vi "Odom_Begin.vi"   [LabVIEW 2020]
uses:
  <vilib>/Rock Robotics/WPI/ThirdParty/JAS_Junk/TrajLib/Rotation2d_CreateAngle.vi
  <vilib>/Rock Robotics/WPI/ThirdParty/JAS_Junk/TrajLib/Translation2d_Create.vi
  Robot Global Data.vi
  <vilib>/Rock Robotics/WPI/ThirdParty/JAS_Junk/TrajLib/Trajectory_Library.lvlib
types:
  T1 = typedef "Trajectory_Library.lvlib/ROTATION2D.ctl" = cluster{"VALUE":dbl, "COS":dbl, "SIN":dbl}
  T2 = typedef "Trajectory_Library.lvlib/SWERVE_DRIVE_MODULE_STATE.ctl" = cluster{"Speed":dbl, "Angle":T1}
  T3 = typedef "Trajectory_Library.lvlib/SWERVE_DRIVE_MODULE_POSITION.ctl" = cluster{"Distance":dbl, "Angle":T1, "P":bool}
  T4 = typedef "Trajectory_Library.lvlib/POSE2D.ctl" = cluster{"TRANSLATION":T5, "ROTATION":T1}
  T5 = typedef "Trajectory_Library.lvlib/TRANSLATION2D.ctl" = cluster{"X":dbl, "Y":dbl}
  T6 = typedef "Trajectory_Library.lvlib/SWERVE_DRIVE_ODOMETRY.ctl" = cluster{"POSE":T4, "GyroOffset":T1, "PreviousAngle":T1, "PrevModulePositions":T3[], "NumModules":i32}
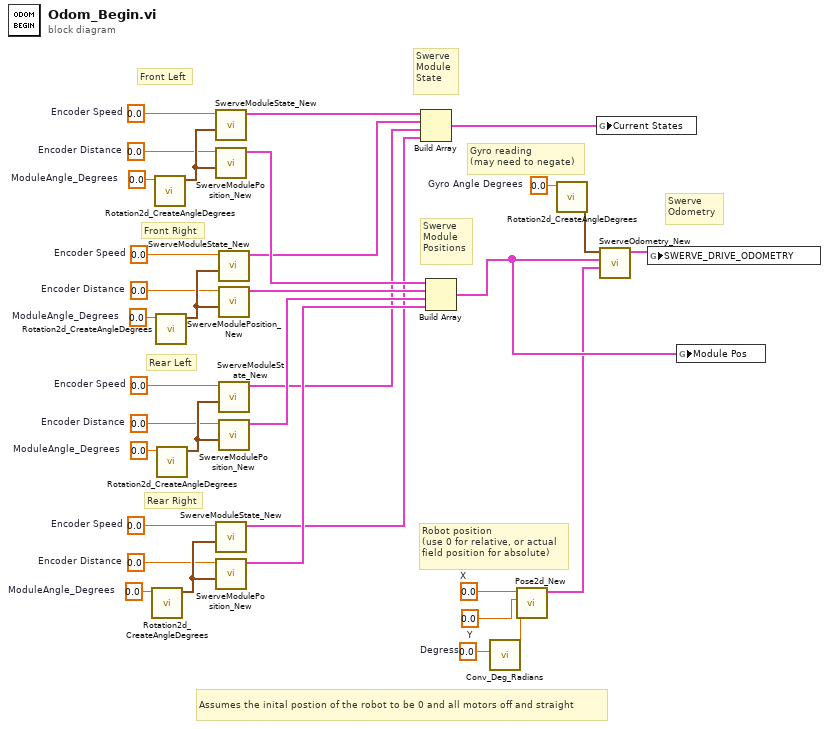
[diagram p0: block diagram]
diagram:
  w18 = 0.0  # Encoder Distance
  w17 = 0.0  # Encoder Distance
  w16 = 0.0  # Encoder Distance
  w14 = 0.0  # Encoder Distance
  w10 = 0.0  # ModuleAngle_Degrees
  w9 = 0.0  # Encoder Speed
  w8 = 0.0  # ModuleAngle_Degrees
  w7 = 0.0  # Encoder Speed
  w6 = 0.0  # ModuleAngle_Degrees
  w5 = 0.0  # Encoder Speed
  w3 = 0.0  # ModuleAngle_Degrees
  w2 = 0.0  # Encoder Speed
  w32 = 0.0  # Degress
  w31 = 0.0  # X
  w30 = 0.0  # Y
  w27 = 0.0  # Gyro Angle Degrees
  # "Assumes the inital postion of the robot to be 0 and all motors off and straight"
  # "Swerve\nModule\nPositions"
  # "Front Left"
  # "Swerve\nModule\nState"
  # "Rear Right"
  # "Rear Left"
  # "Front Right"
  # "Swerve\nOdometry"
  # "Robot position\n(use 0 for relative, or actual \nfield position for absolute)"
  # "Gyro reading\n(may need to negate)"
  n1 = call <vilib>:"Rotation2d_CreateAngleDegrees.vi"("Angle_Degrees"=w10) -> ("ROTATION"=w25:T1)  [unwired: 10 in]
  n2 = call <vilib>:"Rotation2d_CreateAngleDegrees.vi"("Angle_Degrees"=w3) -> ("ROTATION"=w22:T1)  [unwired: 10 in]
  n3 = call <vilib>:"Rotation2d_CreateAngleDegrees.vi"("Angle_Degrees"=w6) -> ("ROTATION"=w23:T1)  [unwired: 10 in]
  n4 = call <vilib>:"Rotation2d_CreateAngleDegrees.vi"("Angle_Degrees"=w8) -> ("ROTATION"=w24:T1)  [unwired: 10 in]
  n5 = call <vilib>:"SwerveModuleState_New.vi"("ROTATION"=w22, "Speed"=w2) -> ("SWERVE_DRIVE_MODULE_STATE"=w4:T2)  [unwired: 9 in]
  n6 = call <vilib>:"SwerveModulePosition_New.vi"("ROTATION"=w22, "Distance"=w14) -> ("SWERVE_DRIVE_MODULE_POSITION"=w15:T3)  [unwired: 9 in]
  n7 = call <vilib>:"SwerveModuleState_New.vi"("ROTATION"=w25, "Speed"=w9) -> ("SWERVE_DRIVE_MODULE_STATE"=w13:T2)  [unwired: 9 in]
  n8 = call <vilib>:"SwerveModulePosition_New.vi"("ROTATION"=w25, "Distance"=w18) -> ("SWERVE_DRIVE_MODULE_POSITION"=w21:T3)  [unwired: 9 in]
  n9 = call <vilib>:"SwerveModuleState_New.vi"("ROTATION"=w23, "Speed"=w5) -> ("SWERVE_DRIVE_MODULE_STATE"=w11:T2)  [unwired: 9 in]
  n10 = call <vilib>:"SwerveModulePosition_New.vi"("ROTATION"=w23, "Distance"=w16) -> ("SWERVE_DRIVE_MODULE_POSITION"=w19:T3)  [unwired: 9 in]
  n11 = call <vilib>:"SwerveModuleState_New.vi"("ROTATION"=w24, "Speed"=w7) -> ("SWERVE_DRIVE_MODULE_STATE"=w12:T2)  [unwired: 9 in]
  n12 = call <vilib>:"SwerveModulePosition_New.vi"("ROTATION"=w24, "Distance"=w17) -> ("SWERVE_DRIVE_MODULE_POSITION"=w20:T3)  [unwired: 9 in]
  n13 = Build Array(w4, w11, w12, w13) -> (w1:T2[])
  n14 = Build Array(w15, w19, w20, w21) -> (w34:T3[])
  n15 = call <vilib>:"Conv_Deg_Radians.vi"("Degress"=w32) -> ("Radians"=w29:dbl)  [unwired: 10 in]
  n16 = call <vilib>:"Pose2d_New.vi"("Heading"=w29, "Y"=w30, "X"=w31) -> ("out POSe"=w33:T4)  [unwired: 8 in]
  n17 = call <vilib>:"Rotation2d_CreateAngleDegrees.vi"("Angle_Degrees"=w27) -> ("ROTATION"=w28:T1)  [unwired: 10 in]
  n18 = global write "Robot Global Data.vi" "Current States"(w1) -> ()
  n19 = call <vilib>:"SwerveOdometry_New.vi"("InitialPose"=w33, "Module Positions"=w34, "gyroAngle"=w28) -> ("SWERVE_DRIVE_ODOMETRY"=w26:T6)  [unwired: 8 in]
  n20 = global write "Robot Global Data.vi" "SWERVE_DRIVE_ODOMETRY"(w26) -> ()
  n21 = global write "Robot Global Data.vi" "Module Pos"(w34) -> ()
